vi "scrollbar_index-page.vi"(8 "error in (no error)":errorcluster, 9 "seek":i32, 10 "data_display":i32, 11 "data_available":i32) -> (0 "error out":errorcluster, 2 "length":i32=-1, 3 "index":i32=-1)   [LabVIEW 2015, in "lv-graph.lvlib"]
doc: "This VI will relegate scrollbar values with the data available and what's visible on the graph."
uses:
  lv-graph.lvlib
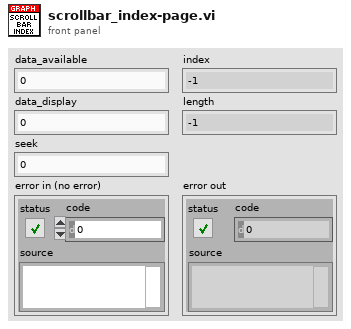
[diagram p1: front panel]
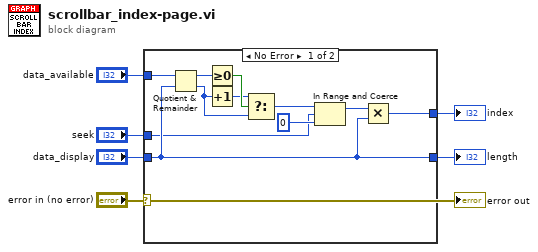
[diagram p0: block diagram]
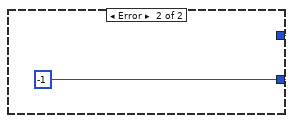
[diagram p2: hidden frame]
diagram:
  n1 = case shown="No Error" "error in (no error)" {
    tunnel: "seek" -> [w8 _]
    tunnel: "data_display" -> [w12 _]
    tunnel: [w9 w18] -> w4
    tunnel: [w12 w18] -> w3
    tunnel: "data_available" -> [w17 _]
    frame No Error {
      n2 = Quotient & Remainder(x=w17, y=w12) -> (x-y*floor(x/y)=w16:i32, floor(x/y)=w14:i32)
      n3 = Greater Or Equal To 0?(x=w16) -> (x >= 0?=w15:bool)
      n4 = Increment(x=w14) -> (x+1=w13:i32)
      n5 = Select(t=w13, s=w15, f=w14) -> (s? t:f=w11:i32)
      n6 = In Range and Coerce(upper limit=w11, x=w8, lower limit=0) -> (coerced(x)=w7:i32)  [unwired: 1 out]
      n7 = Multiply(x=w7, y=w12) -> (x*y=w9:i32)
    }
    frame Error {
      w18 = -1 ("Seek")
    }
  }
  "index" <- w4
  "length" <- w3
  "error out" <- "error in (no error)"
